vi "Constructor.vi"(8 "error in (no error)":errorcluster, 10 "Turkey.lvclass":refnum<class "Turkey.lvclass">, 11 "TurkeyAdapter in":refnum<class "TurkeyAdapter.lvclass">) -> (0 "error out":errorcluster, 3 "TurkeyAdapter out":refnum<class "TurkeyAdapter.lvclass">)   [LabVIEW 2013, in "TurkeyAdapter.lvclass"]
uses:
  TurkeyAdapter.lvclass
  Turkey.lvclass/Turkey.lvclass
  TurkeyAdapter.lvclass/TurkeyAdapter.ctl
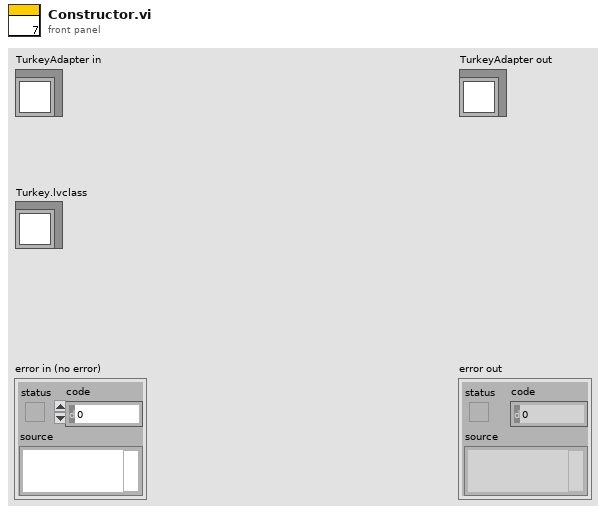
[diagram p1: front panel]
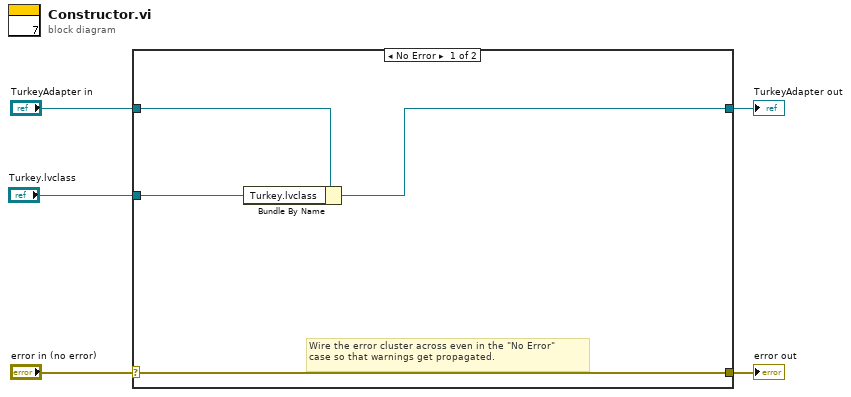
[diagram p0: block diagram]
diagram:
  n1 = case shown="No Error" "error in (no error)" {
    selector: "error in (no error)" -> [w9 w11]
    tunnel: [w9 w11] -> w4
    tunnel: [w7 w10] -> w2
    tunnel: "TurkeyAdapter in" -> [w8 w10]
    tunnel: "Turkey.lvclass" -> [w6 _]
    frame No Error {
      # "Wire the error cluster across even in the \"No Error\"\ncase so that warnings get propagated."
      n2 = Bundle By Name(cluster=w8, "Turkey.lvclass"=w6) -> (w7:refnum<class "TurkeyAdapter.lvclass">)
    }
    frame Error {
    }
  }
  "error out" <- w4
  "TurkeyAdapter out" <- w2
